vi "Make Status Message.vi"(10 "Direction":enum16{"Rising", "Falling"}(ring), 11 "TTrigger":dbl) -> (3 "Status Message":string)   [LabVIEW 2024]
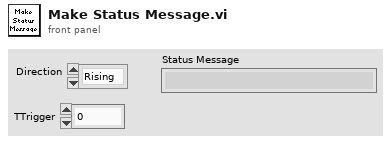
[diagram p1: front panel]
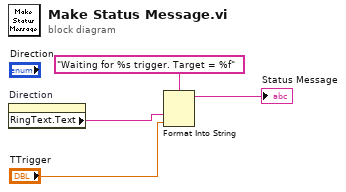
[diagram p0: block diagram]
diagram:
  n1 = property on="Direction" class="Enum (strict)"() -> ("RingText.Text"=w3:string)  [unwired: 2 in, 2 out]
  n2 = Format Into String(format string="Waiting for %s trigger. Target = %f", w3, "TTrigger") -> (resulting string=→"Status Message":string)  [unwired: 2 in, 1 out]
